vi "GetGearIntakeSpeed.vi"() -> (2 "Gear Intake Speed":dbl)   [LabVIEW 2016, in "Gear Intake.lvclass"]
uses:
  Gear Intake.lvclass
  Gear Intake.lvclass/Gear Intake.ctl
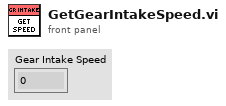
[diagram p1: front panel]
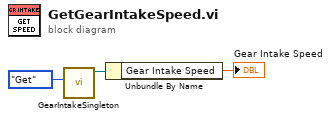
[diagram p0: block diagram]
diagram:
  n1 = call "GearIntakeSingleton.vi"("Get/Set"=enum16{"Get", "Set"}."Get") -> ("Gear Intake.lvclass"=w1:refnum<class "Gear Intake.lvclass">)  [unwired: 9 in, 1 out]
  n2 = Unbundle By Name(w1) -> ("Gear Intake Speed"=→"Gear Intake Speed":dbl)
